vi "Test Invalid Registration - Empty Asset Name.vi"() -> (2 "Success":bool)   [LabVIEW 2024]
uses:
  Mock Sift Proxy Server/Mock Sift Proxy Server.lvclass
  Sift API/Sift Client.lvclass
  Sift API/Types/Data Type.ctl
  Sift Client.lvlib
panel:
  out "Server Error":errorcluster
  out "Error":errorcluster
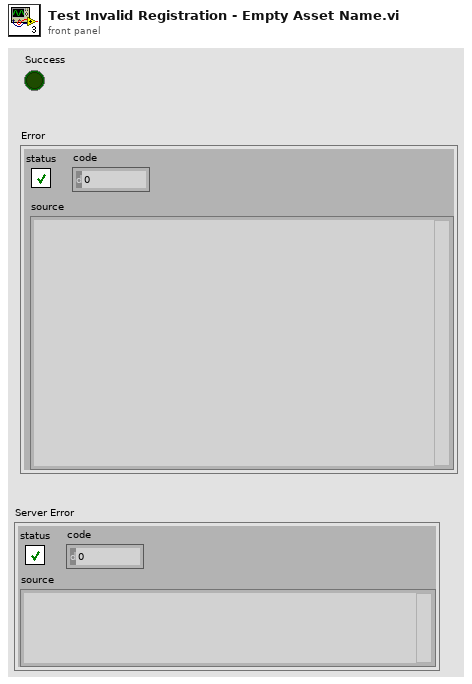
[diagram p1: front panel]
types:
  T1 = typedef "Sift Client.lvlib/Data Type.ctl" = enum8{"double", "float", "uint64", "int64", "uint32", "int32", "bool", "bit field", "enum"}
  T2 = typedef "Sift Client.lvlib/Channel Config.ctl" = cluster{"name":string, "data_type":T1, "description":string, "component":string, "unit":string, "bit_field_elements":T3[], "enum_types":T4[]}
  T3 = typedef "Sift Client.lvlib/Bit Field.ctl" = cluster{"index":u32, "bit_count":u32, "name":string}
  T4 = typedef "Sift Client.lvlib/Enum.ctl" = cluster{"Key":u32, "Name":string}
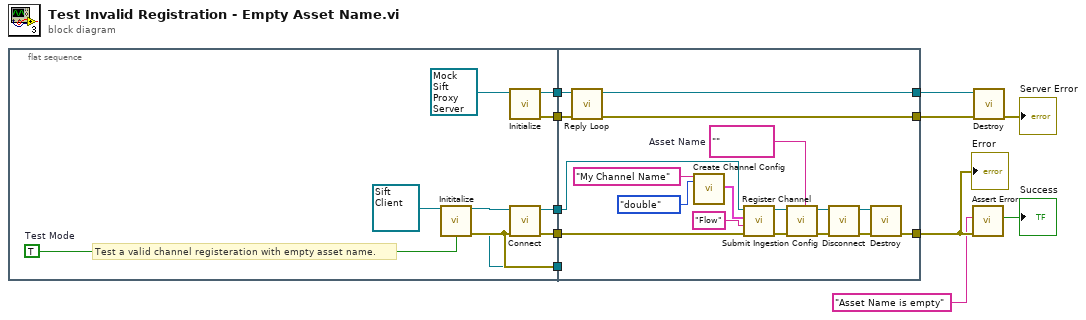
[diagram p0: block diagram]
diagram:
  n1 = flat-sequence {
    tunnel: [w20] -> w10
    tunnel: [w17] -> w8
    tunnel: [w16] -> w7
    tunnel: [w15] -> w6
    tunnel: [w14] -> w5
    tunnel: [w13] -> w4
    tunnel: [w28] -> w11
    tunnel: w10 -> [w29]
    tunnel: [w37] -> w9
    tunnel: w8 -> [_]
    tunnel: w7 -> [_]
    tunnel: w6 -> [w27]
    tunnel: w5 -> [w26]
    tunnel: w4 -> [w23]
    tunnel: [w22] -> w3
    frame #0 {
      w18 = TRUE  # Test Mode
      # "Test a valid channel registeration with empty asset name."
      n2 = call-dynamic "Inititalize.vi"("Sift Client in"=refnum<class "Sift Client.lvclass"> refnum ("Sift Client.lvlib:Sift Client.lvclass"), "Test Mode"=w18) -> ("Sift Client out"=w16:refnum<class "Sift Client.lvclass">, "error out"=w17:errorcluster)  [unwired: 12 in]
      n3 = call-dynamic "Initialize.vi"("Mock Sift Proxy Server in"=refnum<class "Mock Sift Proxy Server.lvclass"> refnum ("Mock Sift Proxy Server.lvclass")) -> ("error out"=w13:errorcluster, "Mock Sift Proxy Server out"=w20:refnum<class "Mock Sift Proxy Server.lvclass">)  [unwired: 9 in]
      n4 = call-dynamic "Connect.vi"("error in (no error)"=w17, "Sift Client in"=w16) -> ("error out"=w15:errorcluster, "Sift Client out"=w14:refnum<class "Sift Client.lvclass">)  [unwired: 7 in, 1 out]
    }
    frame #1 {
      w33 = ""  # Asset Name
      n5 = call-dynamic "Reply Loop.vi"("error in (no error)"=w23, "Mock Sift Proxy Server in"=w29) -> ("error out"=w22:errorcluster, "Mock Sift Proxy Server out"=w28:refnum<class "Mock Sift Proxy Server.lvclass">)  [unwired: 8 in]
      n6 = call "Create Channel Config.vi"("Name"="My Channel Name", "Data Type"=Data_Type."double" ("Enum")) -> ("Output"=w34:T2)  [unwired: 17 in]
      n7 = call-dynamic "Register Channel.vi"("error in (no error)"=w27, "Flow Name"="Flow", "Channel Config"=w34, "Sift Client in"=w26) -> ("error out"=w38:errorcluster, "Sift Client out"=w31:refnum<class "Sift Client.lvclass">)  [unwired: 6 in]
      n8 = call-dynamic "Submit Ingestion Config.vi"("error in (no error)"=w38, "Asset Name"=w33, "Sift Client in"=w31) -> ("error out"=w39:errorcluster, "Sift Client out"=w30:refnum<class "Sift Client.lvclass">)  [unwired: 6 in, 1 out]
      n9 = call-dynamic "Disconnect.vi"("error in (no error)"=w39, "Sift Client in"=w30) -> ("error out"=w24:errorcluster, "Sift Client out"=w25:refnum<class "Sift Client.lvclass">)  [unwired: 8 in]
      n10 = call-dynamic "Destroy.vi"("error in (no error)"=w24, "Sift Client in"=w25) -> ("error out"=w37:errorcluster)  [unwired: 8 in, 1 out]
    }
  }
  n11 = call "Assert Error.vi"("Error"=w9, "Error String"="Asset Name is empty") -> ("Success"=→"Success":bool)  [unwired: 9 in]
  n12 = call-dynamic "Destroy.vi"("error in (no error)"=w3, "Mock Sift Proxy Server in"=w11) -> ("error out"=→"Server Error":errorcluster)  [unwired: 8 in, 1 out]
  "Error" <- w9
